vi "Get_DXF.vi"(7 "Save as":string="PartStudio1", 8 "error in":errorcluster, 9 "Part Id":string="JHK", 10 "microversion":string="6ece3c470dc3e0fb2626e5c7", 11 "Device In":T1) -> (0 "error out":errorcluster, 2 "Comm":T2, 3 "Device Out":T1, 4 "DXF Text":string)   [LabVIEW 2019]
uses:
  <userlib>/Onshape/_SubVI/Cluster.ctl
  <userlib>/IoT Devices/_subVIs/HTTPComm.ctl
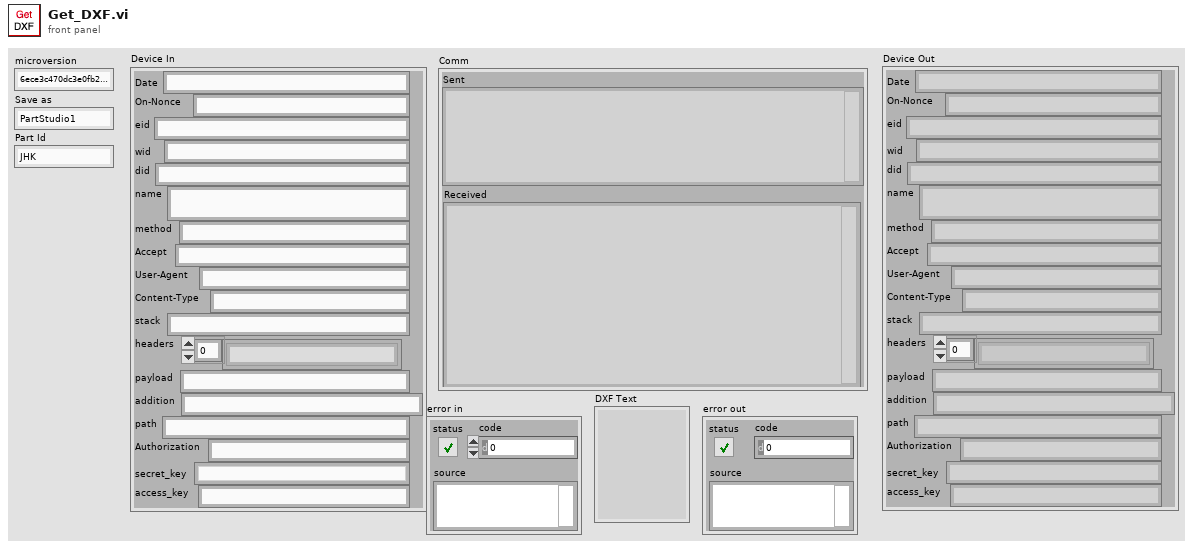
[diagram p1: front panel]
types:
  T1 = typedef "Cluster.ctl" = cluster{"Date":string, "On-Nonce":string, "eid":string, "wid":string, "did":string, "name":string, "method":string, "Accept":string, "User-Agent":string, "Content-Type":string, "stack":string, "headers":string[], "payload":string, "addition":string, "path":string, "Authorization":string, "secret_key":string, "access_key":string}
  T2 = typedef "HTTPComm.ctl" = cluster{"url":string, "sent headers":string, "sent body":string, "headers":string, "body":string, "Sent":string, "Received":string}
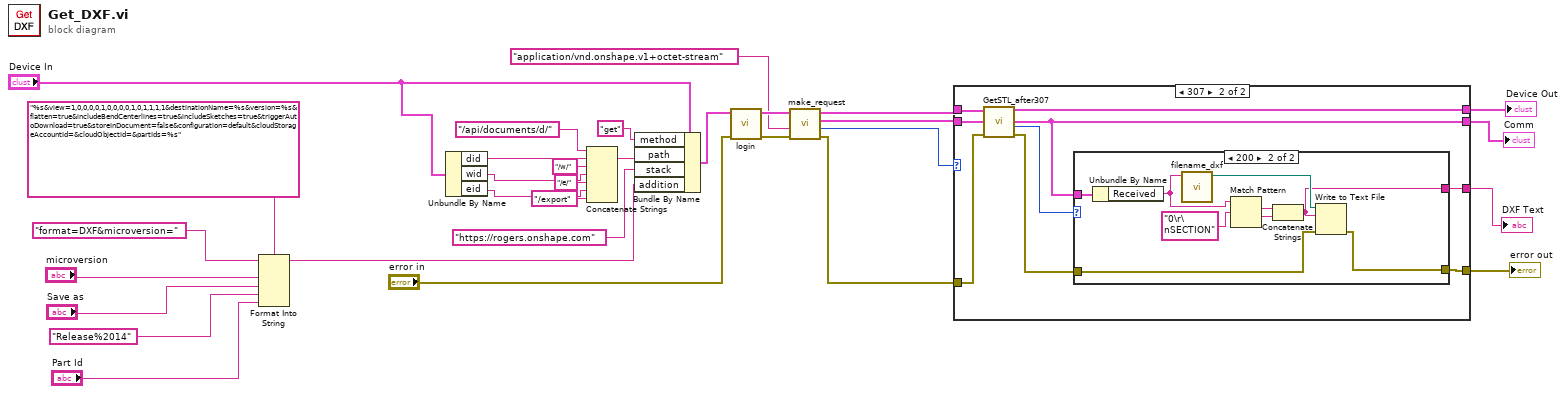
[diagram p0: block diagram]
diagram:
  n1 = Format Into String(format string="%s&view=1,0,0,0,0,1,0,0,0,0,1,0,1,1,1,1&destinationName=%s&version=%s&flatten=true&includeBendCenterlines=true&includeSketches=true&triggerAutoDownload=true&storeInDocument=false&configuration=default&cloudStorageAccountId=&cloudObjectId=&partIds=%s", initial string="format=DXF&microversion=", "microversion", "Save as", "Release%2014" ("input 3"), "Part Id") -> (resulting string=w4:string)  [unwired: 1 in, 1 out]
  n2 = Unbundle By Name("Device In") -> ("did"=w24:string, "wid"=w20:string, "eid"=w18:string)
  n3 = Concatenate Strings("/api/documents/d/" ("payload"), w24, "/w/" ("string"), w20, "/e/" ("string"), w18, "/export" ("string")) -> (w29:string)
  n4 = Bundle By Name(cluster="Device In", "method"="get" ("Method"), "path"=w29, "stack"="https://rogers.onshape.com" ("stacks"), "addition"=w4) -> (w26:T1)
  n5 = call <userlib>:"login.vi"("error in"="error in", "Device In"=w26) -> ("error out"=w27:errorcluster, "Device Out"=w25:T1)  [unwired: 8 in]
  n6 = call <userlib>:"make_request.vi"("Error in"=w27, "Accept"="application/vnd.onshape.v1+octet-stream", "Device In"=w25) -> ("error out"=w15:errorcluster, "error"=w16:i32, "Comm"=w14:T2, "Device Out"=w13:T1)  [unwired: 4 in, 1 out]
  n7 = case shown="307" w16 {
    tunnel: w15 -> [w32 w43]
    tunnel: w14 -> [w33 w42]
    tunnel: w13 -> [w34 w41]
    tunnel: [w34 w40] -> w12
    tunnel: [w33 w39] -> w11
    tunnel: [w32 w36] -> w10
    tunnel: [_ w35] -> w9
    frame 0, Default {
    }
    frame 307 {
      n8 = call <userlib>:"GetSTL_after307.vi"("error in (no error)"=w43, "Comm in"=w42, "Device in"=w41) -> ("error out"=w37:errorcluster, "error"=w38:i32, "Comm out"=w39:T2, "Device Out"=w40:T1)  [unwired: 5 in]
      n9 = case shown="200" w38 {
        tunnel: w39 -> [_ w53]
        tunnel: [w44 w46] -> w36
        tunnel: w37 -> [w44 w47]
        tunnel: [_ w45] -> w35
        frame 0, Default {
        }
        frame 200 {
          n10 = Unbundle By Name(w53) -> ("Received"=w49:string)
          n11 = call "filename_dxf.vi"("Received"=w49) -> ("appended path"=w48:path)  [unwired: 10 in]
          n12 = Match Pattern(string=w49, regular expression="0\r\nSECTION") -> (match substring=w51:string, after substring=w50:string)  [unwired: 1 in, 2 out]
          n13 = Concatenate Strings(w51, w50) -> (w45:string)
          n14 = Write to Text File(file (use dialog)=w48, text=w45, error in=w47) -> (error out=w46:errorcluster)  [unwired: 1 in, 2 out]
        }
      }
    }
  }
  "Device Out" <- w12
  "Comm" <- w11
  "error out" <- w10
  "DXF Text" <- w9
